vi "set_number_of_pixels.vi"(8 "error in (no error)":errorcluster, 10 "number of pixels":i64, 11 "FPGAWrapperDL090211Galvo in":refnum<class "FPGAWrapperDL090211Galvo_grabber.lvclass">) -> (0 "error out":errorcluster, 3 "FPGAWrapperDL090211Galvo out":refnum<class "FPGAWrapperDL090211Galvo_grabber.lvclass">)   [LabVIEW 2010, in "FPGAWrapperDL090211Galvo_grabber.lvclass"]
uses:
  FPGAWrapperDL090211Galvo_grabber.lvclass
  FPGAWrapperDL090211Galvo_grabber.lvclass/FPGAWrapperDL090211Galvo_grabber.ctl
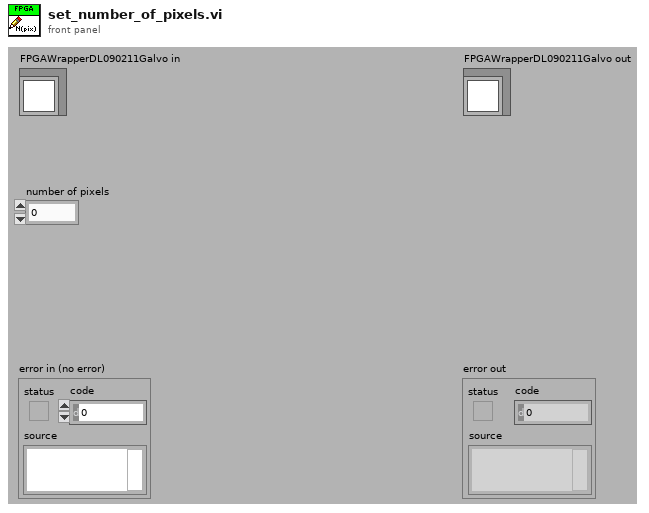
[diagram p1: front panel]
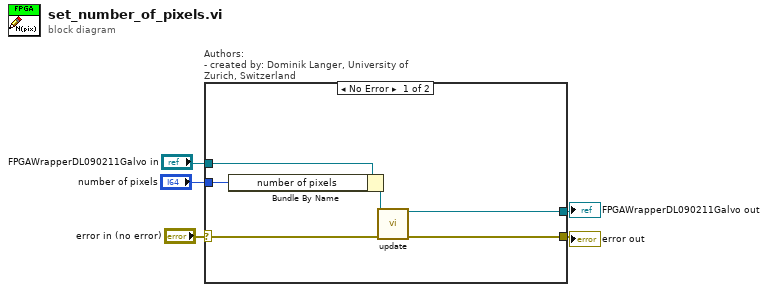
[diagram p0: block diagram]
diagram:
  n1 = case "Authors: \n- created by: Dominik Langer, University of Zurich, Switzerland" shown="No Error" "error in (no error)" {
    selector: "error in (no error)" -> [w7 w13]
    tunnel: [w8 w12] -> w1
    tunnel: [w6 w13] -> w2
    tunnel: "FPGAWrapperDL090211Galvo in" -> [w11 w12]
    tunnel: "number of pixels" -> [w10 _]
    frame No Error {
      n2 = Bundle By Name(cluster=w11, "number of pixels"=w10) -> (w9:refnum<class "FPGAWrapperDL090211Galvo_grabber.lvclass">)
      n3 = call-dynamic "update.vi"("error in (no error)"=w7, "FPGAWrapperDL120115Galvo in"=w9) -> ("error out"=w6:errorcluster, "FPGAWrapperDL120115Galvo out"=w8:refnum<class "FPGAWrapperDL090211Galvo_grabber.lvclass">)  [unwired: 8 in]
    }
    frame Error {
    }
  }
  "error out" <- w2
  "FPGAWrapperDL090211Galvo out" <- w1
